vi "exnSpectralBlock spectral measurements peak DDT.vi"(0 "Signals":dynamicdata(graph), 5 "Restart Averaging":bool, 7 "View":T2, 9 "Spectrum Window":u16, 11 "error in (no error)":errorcluster, 12 "Spectrum Averaging Parameters":T1={"averaging mode"=0, "weighting mode"=1, "number of averages"=10} {"averaging mode" items=["No averaging", "Vector averaging", "RMS averaging", "Peak hold"]; "weighting mode" items=["Linear", "Exponential"]}, 14 "All Spectra":bool) -> (4 "Measurement Output":dynamicdata(graph), 6 "averaging done":bool, 10 "Phase":dynamicdata(graph), 15 "error out":errorcluster)   [LabVIEW 2020]
uses:
  <vilib>/measure/NI_MAPro.lvlib
panel:
  in  "measurement":string="FFT - (Peak)"
  in  "string":string=" Phase"
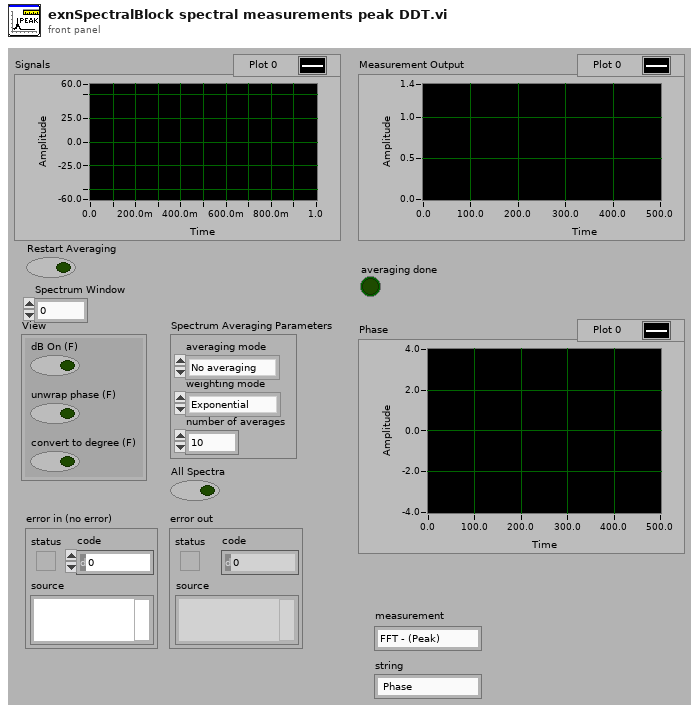
[diagram p1: front panel]
types:
  T1 = cluster{"averaging mode":u16, "weighting mode":u16, "number of averages":u32}
  T2 = cluster{"dB On (F)":bool, "unwrap phase (F)":bool, "convert to degree (F)":bool}
  T3 = enum16{"None ", "Hanning", "Hamming", "Blackman-Harris", "Exact Blackman", "Blackman", "Flat Top", "4 Term B-Harris ", "7 Term B-Harris", "Low Sidelobe"}
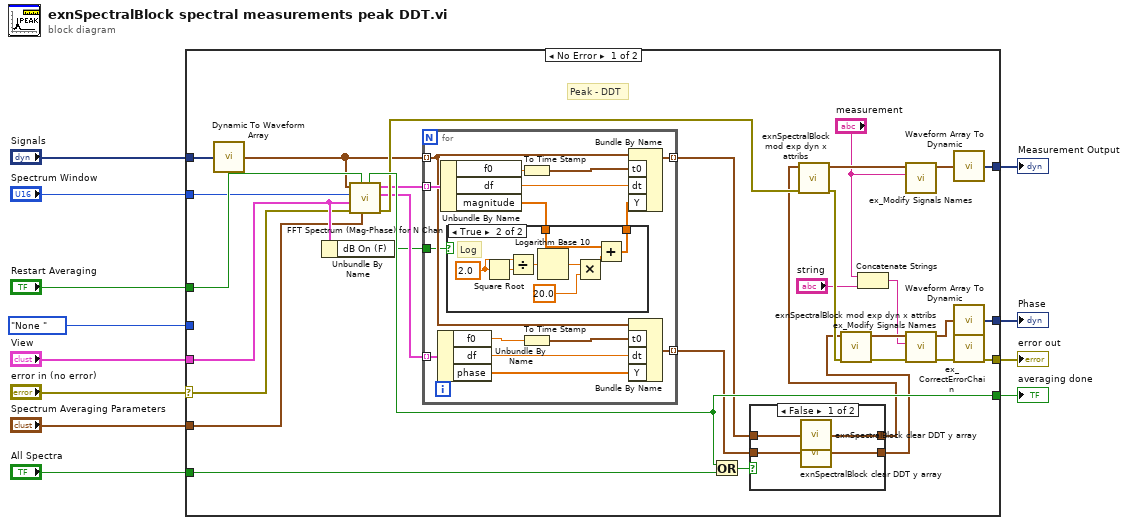
[diagram p0: block diagram]
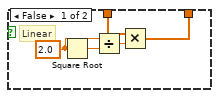
[diagram p2: hidden frame]
diagram:
  n1 = case shown="No Error" "error in (no error)" {
    selector: "error in (no error)" -> [w18 w78]
    tunnel: [w43 _] -> w12
    tunnel: [w42 _] -> w11
    tunnel: [w41 _] -> w10
    tunnel: "All Spectra" -> [w40 _]
    tunnel: "Spectrum Averaging Parameters" -> [w13 _]
    tunnel: "Restart Averaging" -> [w39 _]
    tunnel: T3."None " ("window") -> [_ _]
    tunnel: "Spectrum Window" -> [w19 _]
    tunnel: "View" -> [w37 _]
    tunnel: "Signals" -> [w35 _]
    tunnel: [w34 w78] -> w3
    frame No Error {
      # "Peak - DDT"
      n2 = call <vilib>:"Dynamic To Waveform Array.vi"("Input"=w35) -> ("Output"=w20:waveform(dbl)[])  [unwired: 4 in]
      n3 = Unbundle By Name(w37) -> ("dB On (F)"=w14:bool)
      n4 = call <vilib>:"FFT Spectrum (Mag-Phase) for N Chan.vi"("averaging parameters"=w13, "restart averaging (F)"=w39, "error in (no error)"=w18, "view"=w37, "window"=w19, "time signals"=w20) -> ("error out"=w36:errorcluster, "phases"=w15:cluster{"f0":dbl, "df":dbl, "phase":dbl[]}[], "magnitudes"=w16:cluster{"f0":dbl, "df":dbl, "magnitude":dbl[]}[], "averaging done"=w41:bool)  [unwired: 1 in, 1 out]
      n5 = for {
        tunnel: w20 -> [w47] mode=indexing
        tunnel: [w56] -> w23 mode=indexing
        tunnel: w16 -> [w55] mode=indexing
        tunnel: [w46] -> w24 mode=indexing
        tunnel: w15 -> [w45] mode=indexing
        tunnel: w14 -> [w44]
        n6 = Unbundle By Name(w45) -> ("f0"=w50:dbl, "df"=w49:dbl, "phase"=w48:dbl[])
        n7 = Unbundle By Name(w55) -> ("f0"=w57:dbl, "df"=w58:dbl, "magnitude"=w54:dbl[])
        n8 = case shown="True" w44 {
          tunnel: w54 -> [w62 w71]
          tunnel: [w61 w70] -> w53
          frame False {
            w60 = 2.0 ("y")
            # "Linear"
            n9 = Square Root(x=w60) -> (sqrt(x)=w63:dbl)
            n10 = Divide(x=w60, y=w63) -> (x/y=w59:dbl)
            n11 = Multiply(x=w62, y=w59) -> (x*y=w61:dbl[])
          }
          frame True {
            w68 = 2.0 ("y")
            # "Log"
            n12 = Square Root(x=w68) -> (sqrt(x)=w69:dbl)
            n13 = Divide(x=w68, y=w69) -> (x/y=w66:dbl)
            n14 = Logarithm Base 10(1:w66) -> (0:w64:dbl)
            n15 = Multiply(x=w64, y=20.0) -> (x*y=w65:dbl)
            n16 = Add(x=w71, y=w65) -> (x+y=w70:dbl[])
          }
        }
        n17 = To Time Stamp(1:w57) -> (0:w52:timestamp)
        n18 = To Time Stamp(1:w50) -> (0:w51:timestamp)
        n19 = Bundle By Name(cluster=w47, "t0"=w52, "dt"=w58, "Y"=w53) -> (w56:waveform(dbl))
        n20 = Bundle By Name(cluster=w47, "t0"=w51, "dt"=w49, "Y"=w48) -> (w46:waveform(dbl))
      }
      n21 = Or(x=w41, y=w40) -> (x .or. y?=w25:bool)
      n22 = case shown="False" w25 {
        tunnel: w24 -> [w73 w76]
        tunnel: w23 -> [w75 w77]
        tunnel: [w74 w77] -> w22
        tunnel: [w72 w76] -> w21
        frame False {
          n23 = call <vilib>:"exnSpectralBlock clear DDT y array.vi"("Array In"=w75) -> ("Array Out"=w74:waveform(dbl)[])
          n24 = call <vilib>:"exnSpectralBlock clear DDT y array.vi"("Array In"=w73) -> ("Array Out"=w72:waveform(dbl)[])
        }
        frame True {
        }
      }
      n25 = call <vilib>:"exnSpectralBlock mod exp dyn x attribs.vi"("error in (no error)"=w36, "Signals in"=w22) -> ("error out"=w38:errorcluster, "Signals out"=w33:waveform(dbl)[])  [unwired: 8 in]
      n26 = call <vilib>:"exnSpectralBlock mod exp dyn x attribs.vi"("error in (no error)"=w38, "Signals in"=w21) -> ("error out"=w31:errorcluster, "Signals out"=w28:waveform(dbl)[])  [unwired: 8 in]
      n27 = Concatenate Strings("measurement", "string") -> (w26:string)
      n28 = call <vilib>:"ex_Modify Signals Names.vi"("Name Modifier"="measurement", "Array of Waveforms In"=w33) -> ("Array of Waveforms Out"=w32:waveform(dbl)[])  [unwired: 8 in, 1 out]
      n29 = call <vilib>:"ex_Modify Signals Names.vi"("error in (no error)"=w31, "Name Modifier"=w26, "Array of Waveforms In"=w28) -> ("error out"=w30:errorcluster, "Array of Waveforms Out"=w29:waveform(dbl)[])  [unwired: 7 in]
      n30 = call <vilib>:"Waveform Array To Dynamic.vi"("Input"=w32) -> ("Output"=w43:dynamicdata)  [unwired: 4 in]
      n31 = call <vilib>:"Waveform Array To Dynamic.vi"("Input"=w29) -> ("Output"=w42:dynamicdata)  [unwired: 4 in]
      n32 = call <vilib>:"ex_CorrectErrorChain.vi"("error in (no error)"=w30) -> ("error out"=w34:errorcluster)  [unwired: 10 in]
    }
    frame Error {
    }
  }
  "Phase" <- w11
  "Measurement Output" <- w12
  "averaging done" <- w10
  "error out" <- w3
